vi "2_Analog_Meter_Reader(Evaluation).vi"() -> ()   [LabVIEW 2020]
uses:
  Controls/Regression_Report.ctl
  <vilib>/Ngene/DeepLTK/Toolkit/NN_Network/Controls/NN_Save_Before_Destroy_Options.ctl
  <vilib>/Ngene/DeepLTK/Toolkit/NN_Network/subVIs/NN_Predict/NN_Predict(In3D_Out1D).vi
  <vilib>/Ngene/DeepLTK/Toolkit/NN_Train/Eval_Loss/NN_Eval_Test_Error_Loss/NN_Eval(In3D_Out1D).vi
  <vilib>/Ngene/DeepLTK/Toolkit/Deep_Learning_Toolkit_by_Ngene.lvlib
panel:
  in  "Image Folder(Test)":path=path "D:/DeepLTK_Examples/Analog_Meter/Test/Images"
  in  "Labels (Test)":path=path "D:/DeepLTK_Examples/Analog_Meter/Test/Labels.csv"
  in  "NN Device":enum16{"CPU", "GPU"}(ring)=enum."GPU"
  in  "Image Folder(Train)":path=path "D:/DeepLTK_Examples/Analog_Meter/Train/Images"
  in  "Labels (Train)":path=path "D:/DeepLTK_Examples/Analog_Meter/Train/Labels.csv"
  out "Metrics (Test)":T1={"Graphs"=[{"Best Linear Fit"=[0.0, 0.7035179734230042, 1.407034993171692, 2.110553026199341, 2.814069986343384, 3.517587900161743, 4.221106052398682, 4.924623012542725, 5.628140926361084, 6.331657886505127, 7.035175800323486, 7.7386932373046875, 8.442211151123047, 9.145729064941406, 9.84924602508545, 10.552763938903809, 11.256280899047852, 11.959798812866211, 12.66331672668457, 13.366833686828613, 14.070351600646973, 14.773868560791016, 15.477387428283691, 16.180904388427734, 16.884422302246094, 17.587940216064453, 18.29145622253418, 18.99497413635254, 19.6984920501709, 20.402009963989258, 21.105527877807617, 21.809045791625977, 22.512563705444336, 23.216079711914062, 23.919597625732422, 24.62311553955078, 25.32663345336914, 26.0301513671875, 26.733667373657227, 27.437185287475586, 28.140703201293945, 28.844221115112305, 29.547739028930664, 30.251256942749023, 30.954774856567383, 31.65829086303711, 32.36180877685547, 33.06532669067383, 33.76884460449219, 34.47236251831055, 35.175880432128906, 35.879398345947266, 36.582916259765625, 37.28643035888672, 37.98994827270508, 38.69346618652344, 39.3969841003418, 40.100502014160156, 40.804019927978516, 41.507537841796875, 42.211055755615234, 42.914573669433594, 43.61809158325195, 44.32160949707031, 45.02512741088867, 45.728641510009766, 46.432159423828125, 47.135677337646484, 47.839195251464844, 48.5427131652832, 49.24623107910156, 49.94974899291992, 50.65326690673828, 51.35678482055664, 52.060302734375, 52.76382064819336, 53.46733856201172, 54.17085266113281, 54.87437057495117, 55.57788848876953, 56.28140640258789, 56.98492431640625, 57.68844223022461, 58.39196014404297, 59.09547805786133, 59.79899597167969, 60.50251388549805, 61.206031799316406, 61.909549713134766, 62.61306381225586, 63.31658172607422, 64.02010345458984, 64.72361755371094, 65.42713928222656, 66.13065338134766, 66.83416748046875, 67.53768920898438, 68.24120330810547, 68.9447250366211, 69.64823913574219, 70.35176086425781, 71.0552749633789, 71.75879669189453, 72.46231079101562, 73.16583251953125, 73.86934661865234, 74.57286071777344, 75.27638244628906, 75.97989654541016, 76.68341827392578, 77.38693237304688, 78.0904541015625, 78.7939682006836, 79.49748992919922, 80.20100402832031, 80.90452575683594, 81.60803985595703, 82.31156158447266, 83.01507568359375, 83.71858978271484, 84.42211151123047, 85.12562561035156, 85.82914733886719, 86.53266143798828, 87.2361831665039, 87.939697265625, 88.64321899414062, 89.34673309326172, 90.05024719238281, 90.75376892089844, 91.45728302001953, 92.16080474853516, 92.86431884765625, 93.56784057617188, 94.27135467529297, 94.9748764038086, 95.67839050292969, 96.38191223144531, 97.0854263305664, 97.78894805908203, 98.49246215820312, 99.19597625732422, 99.89949798583984, 100.60301208496094, 101.30653381347656, 102.01004791259766, 102.71356964111328, 103.41708374023438, 104.12060546875, 104.8241195678711, 105.52764129638672, 106.23115539550781, 106.9346694946289, 107.63819122314453, 108.34170532226562, 109.04522705078125, 109.74874114990234, 110.45226287841797, 111.15577697753906, 111.85929870605469, 112.56281280517578, 113.2663345336914, 113.9698486328125, 114.67337036132812, 115.37688446044922, 116.08039855957031, 116.78392028808594, 117.48743438720703, 118.19095611572266, 118.89447021484375, 119.59799194335938, 120.30150604248047, 121.0050277709961, 121.70854187011719, 122.41206359863281, 123.1155776977539, 123.819091796875, 124.52261352539062, 125.22612762451172, 125.92964935302734, 126.63316345214844, 127.33668518066406, 128.0402069091797, 128.74371337890625, 129.44723510742188, 130.1507568359375, 130.85427856445312, 131.5577850341797, 132.2613067626953, 132.96482849121094, 133.6683349609375, 134.37185668945312, 135.07537841796875, 135.77890014648438, 136.48240661621094, 137.18592834472656, 137.8894500732422, 138.5929718017578, 139.29647827148438, 140.0], "Array 3"=[1.1191103, 1.1208215, 2.0494566, 2.6667647, 3.113812, 4.3983607, 4.9721265, 5.639334, 6.3064847, 6.8345547, 7.8277693, 8.990467, 9.59511, 9.686706, 10.213453, 11.142547, 11.742723, 12.225249, 13.245596, 14.0788765, 14.814651, 15.36693, 15.76402, 16.432852, 17.134659, 17.87731, 18.427813, 19.16861, 20.000216, 20.941538, 21.51821, 22.116674, 22.470608, 23.3825, 24.453438, 25.066845, 25.64973, 26.13289, 26.796333, 27.819569, 28.452826, 29.007662, 29.715298, 30.633392, 31.342394, 32.035053, 32.61452, 33.464294, 34.276417, 34.943382, 35.97995, 36.556244, 37.02365, 37.705124, 38.3015, 39.360004, 39.889103, 40.30833, 40.943993, 41.4772, 42.169846, 42.81026, 43.799282, 44.6952, 45.416332, 46.042446, 46.79732, 47.508343, 48.09876, 48.742836, 49.218735, 49.851227, 50.669456, 51.317608, 51.95643, 52.556763, 53.286587, 53.868534, 54.71111, 55.695065, 56.496944, 57.143272, 57.87432, 58.363266, 59.263767, 59.95194, 60.54199, 61.248116, 62.144474, 62.750816, 63.315197, 63.991894, 64.673294, 65.21437, 65.78511, 66.731705, 67.40204, 68.17529, 68.910904, 69.6694, 70.56884, 71.38461, 72.153244, 72.770386, 73.40299, 73.98696, 74.56206, 75.30551, 76.02788, 76.8059, 77.393326, 78.05725, 78.863556, 79.64017, 80.19238, 80.80632, 81.75397, 82.49788, 83.45299, 83.8592, 84.582375, 85.37528, 86.09314, 86.848175, 87.40028, 88.08168, 88.83669, 89.5325, 90.27479, 90.954704, 91.40349, 91.8369, 92.65036, 93.7729, 94.60417, 95.43445, 96.11843, 96.73094, 97.527145, 98.015366, 98.69766, 99.33419, 99.997765, 100.65184, 101.144066, 102.21565, 102.77403, 103.49586, 103.97933, 104.69403, 105.7315, 106.22682, 106.847534, 107.528824, 108.24076, 108.93027, 109.59428, 110.28842, 110.89985, 111.587975, 112.43388, 113.592705, 114.30132, 114.76443, 115.22754, 115.85933, 117.078224, 118.21052, 118.373405, 118.85284, 119.099075, 120.0473, 120.72142, 121.46607, 122.0247, 122.7984, 123.476135, 124.20413, 124.859024, 125.31311, 125.978096, 126.854614, 127.88554, 128.6452, 129.04144, 129.79903, 130.51143, 130.49928, 131.18375, 132.28572, 133.07285, 133.94731, 134.7844, 135.33304, 136.06282, 136.96729, 137.98709, 138.17464, 138.51686, 138.61647]}, {"Best Linear Fit"=[0.5510894536551477, 0.5528118856345293, 1.4875805447104122, 2.1089659407688175, 2.558965874975776, 3.851998945803168, 4.4295543638213815, 5.101168919513712, 5.77272587681186, 6.304283697222128, 7.304058383959592, 8.47443567437423, 9.083072145866842, 9.17527277535532, 9.705499592873341, 10.640729519089307, 11.244870435915933, 11.73058329446284, 12.757669219775421, 13.59645351485162, 14.337087266320234, 14.893014487322722, 15.292727183514954, 15.965976573628847, 16.67241895833718, 17.419975076813355, 17.97411386767646, 18.719803798181108, 19.556902380254215, 20.50444204328033, 21.084922499749805, 21.687340264617124, 22.043611291943282, 22.96152618089459, 24.039537726424093, 24.656996351959073, 25.243731994036825, 25.730083234785926, 26.397907816141014, 27.427901500386604, 28.065341008863673, 28.623841918112905, 29.336151659242017, 30.260310214122768, 30.973994636926378, 31.671228958351318, 32.254524056349865, 33.10991012857609, 33.92739645742988, 34.598767179920166, 35.6421812900104, 36.222281597078265, 36.69277599990878, 37.37874983527094, 37.9790633388041, 39.044560673224105, 39.577153824769816, 39.99915037969822, 40.63901094067745, 41.1757396569255, 41.87296053872513, 42.5176056063145, 43.51315929073158, 44.41499654791994, 45.14088991034388, 45.771139219280435, 46.53100027470058, 47.24671792081885, 47.84103351157109, 48.48936487638817, 48.968406880915445, 49.60507649085694, 50.428710488316526, 51.08114285879944, 51.72418285113757, 52.328482163548195, 53.06312664199501, 53.64891767040816, 54.49705786464616, 55.48751217123157, 56.2946883875266, 56.94528528918154, 57.681162373263874, 58.17333681166488, 59.07978578028082, 59.77250246765534, 60.36644942868481, 61.07724049215396, 61.97951933703106, 62.5898664808309, 63.15797480222986, 63.839141091624214, 64.5250419690204, 65.06969238441509, 65.64420180735426, 66.59704820243111, 67.2718095503923, 68.05017121002403, 68.79064080606922, 69.55414975978763, 70.45952739827176, 71.28068850467443, 72.05439621405617, 72.67561409478483, 73.31239890151468, 73.90022507318898, 74.47911965387195, 75.22748406981316, 75.95462155755145, 76.7377830833651, 77.32908819804804, 77.99739852586073, 78.80902901797258, 79.59076978339638, 80.14663268619204, 80.76462505684644, 81.71853126237625, 82.46735646547093, 83.42877350160221, 83.83766834180045, 84.5656198868432, 85.36376467493032, 86.086363409207, 86.84638574013086, 87.40214112592403, 88.08803816342727, 88.84803745499346, 89.54844160804494, 90.29563101674482, 90.9800381757852, 91.4317862212556, 91.86805949815552, 92.68689362943319, 93.8168512467299, 94.65360999827732, 95.48937037765891, 96.17787086257923, 96.79442711327201, 97.59588956886408, 98.08733442760543, 98.77413767984383, 99.4148698965217, 100.0828269541834, 100.74122267841074, 101.2366994247449, 102.31536375207514, 102.87743192187078, 103.60402414481081, 104.09069217672791, 104.81011147964568, 105.85443180447106, 106.35302654387701, 106.97783856440267, 107.66362808490345, 108.38026730532866, 109.07432795523411, 109.7427227606916, 110.44145272041884, 111.05691844151508, 111.74958905017425, 112.60108531084664, 113.76756031005539, 114.48085882361796, 114.94702182720592, 115.41319251057976, 116.04915558021928, 117.2761012135343, 118.41587359719979, 118.57983702597413, 119.06243477136897, 119.31029986100326, 120.26478973026079, 120.94336025202396, 121.69293039435007, 122.25524431729423, 123.03405908429353, 123.71626982456907, 124.44907499429496, 125.10829245561264, 125.56537795227734, 126.2347557703289, 127.11706333199626, 128.1547944005271, 128.91947836148685, 129.31833572152544, 130.08092310093693, 130.79803078830147, 130.7858045691629, 131.47478888059436, 132.58404179512874, 133.37636530551043, 134.25660700477312, 135.0992177531695, 135.65148651616815, 136.38608875579257, 137.29652737317892, 138.32306899366648, 138.51185349044076, 138.8563379663706, 138.9566052509644], "Array 3"=[1.1191103, 1.1208215, 2.0494566, 2.6667647, 3.113812, 4.3983607, 4.9721265, 5.639334, 6.3064847, 6.8345547, 7.8277693, 8.990467, 9.59511, 9.686706, 10.213453, 11.142547, 11.742723, 12.225249, 13.245596, 14.0788765, 14.814651, 15.36693, 15.76402, 16.432852, 17.134659, 17.87731, 18.427813, 19.16861, 20.000216, 20.941538, 21.51821, 22.116674, 22.470608, 23.3825, 24.453438, 25.066845, 25.64973, 26.13289, 26.796333, 27.819569, 28.452826, 29.007662, 29.715298, 30.633392, 31.342394, 32.035053, 32.61452, 33.464294, 34.276417, 34.943382, 35.97995, 36.556244, 37.02365, 37.705124, 38.3015, 39.360004, 39.889103, 40.30833, 40.943993, 41.4772, 42.169846, 42.81026, 43.799282, 44.6952, 45.416332, 46.042446, 46.79732, 47.508343, 48.09876, 48.742836, 49.218735, 49.851227, 50.669456, 51.317608, 51.95643, 52.556763, 53.286587, 53.868534, 54.71111, 55.695065, 56.496944, 57.143272, 57.87432, 58.363266, 59.263767, 59.95194, 60.54199, 61.248116, 62.144474, 62.750816, 63.315197, 63.991894, 64.673294, 65.21437, 65.78511, 66.731705, 67.40204, 68.17529, 68.910904, 69.6694, 70.56884, 71.38461, 72.153244, 72.770386, 73.40299, 73.98696, 74.56206, 75.30551, 76.02788, 76.8059, 77.393326, 78.05725, 78.863556, 79.64017, 80.19238, 80.80632, 81.75397, 82.49788, 83.45299, 83.8592, 84.582375, 85.37528, 86.09314, 86.848175, 87.40028, 88.08168, 88.83669, 89.5325, 90.27479, 90.954704, 91.40349, 91.8369, 92.65036, 93.7729, 94.60417, 95.43445, 96.11843, 96.73094, 97.527145, 98.015366, 98.69766, 99.33419, 99.997765, 100.65184, 101.144066, 102.21565, 102.77403, 103.49586, 103.97933, 104.69403, 105.7315, 106.22682, 106.847534, 107.528824, 108.24076, 108.93027, 109.59428, 110.28842, 110.89985, 111.587975, 112.43388, 113.592705, 114.30132, 114.76443, 115.22754, 115.85933, 117.078224, 118.21052, 118.373405, 118.85284, 119.099075, 120.0473, 120.72142, 121.46607, 122.0247, 122.7984, 123.476135, 124.20413, 124.859024, 125.31311, 125.978096, 126.854614, 127.88554, 128.6452, 129.04144, 129.79903, 130.51143, 130.49928, 131.18375, 132.28572, 133.07285, 133.94731, 134.7844, 135.33304, 136.06282, 136.96729, 137.98709, 138.17464, 138.51686, 138.61647]}, {"Best Linear Fit"=[0.0, 140.0], "Array 3"=[0.0, 140.0]}], "y=k*x+b"="y = 0.993*x + 0.572", "R"=0.99997884, "R^2"=0.9999577, "MAE"=0.30468705, "MSE"=0.1540845} {"R" format="%#_7g"}
  out "Metrics (Train)":T1={"Graphs"=[{"Best Linear Fit"=array[1000 elements], "Array 3"=array[1000 elements]}, {"Best Linear Fit"=array[1000 elements], "Array 3"=array[1000 elements]}, {"Best Linear Fit"=[0.0, 140.0], "Array 3"=[0.0, 140.0]}], "y=k*x+b"="y = 0.994*x + 0.559", "R"=0.9999774, "R^2"=0.9999548, "MAE"=0.3035189, "MSE"=0.1533813} {"R" format="%#_7g"}
  in  "Network Configuration File Path":path=path "D:/Ngene/GitHub/deepltk_examples/3_Image_Processing/31_Image_Regression/working/Analog_Meter/Analog_Meter_net_cfg_23_11_30__17_47_53.cfg"
  in  "Weight File Path":path=path "D:/Ngene/GitHub/deepltk_examples/3_Image_Processing/31_Image_Regression/working/Analog_Meter/Analog_Meter_weights_23_11_30__17_47_53.bin"
  # "Overview: Performs evaluation of a trained model over Training and Tests Datasets\nInstructions:\n1. Provide paths to Train and Test datasets \n2. Provide model files (.cfg and .bin).\n2. Run the VI\n3. Drag and drop image on \"Input Image\"\n4. Observe calculated metrics on both train and test datasets."
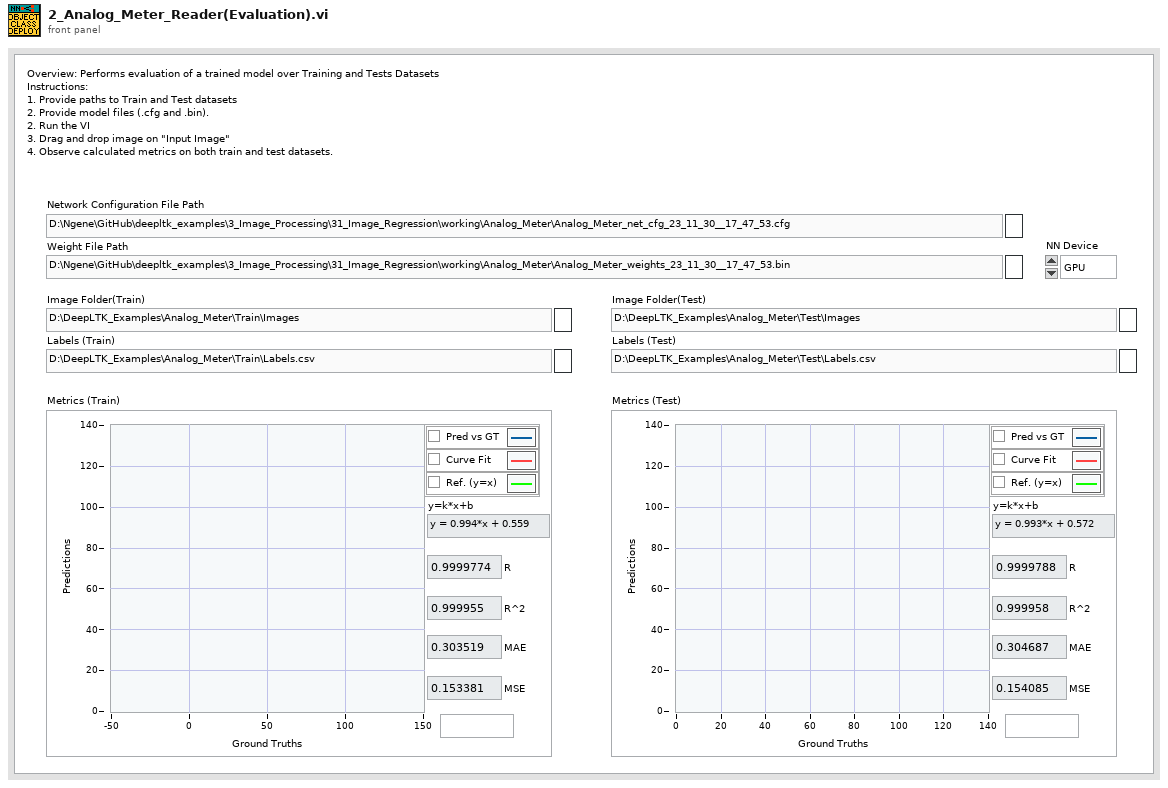
[diagram p1: front panel]
types:
  T1 = typedef "Regression_Report.ctl" = cluster{"Graphs":cluster{"Best Linear Fit":dbl[], "Array 3":sgl[]}[], "y=k*x+b":string, "R":sgl, "R^2":sgl, "MAE":sgl, "MSE":sgl}
  T2 = typedef "Deep_Learning_Toolkit_by_Ngene.lvlib/NN_Save_Before_Destroy_Options.ctl" = cluster{"CFG?":bool, "Weights?":bool, "Render?":bool}
  T3 = typedef "Deep_Learning_Toolkit_by_Ngene.lvlib/NN_Config_Params.ctl" = cluster{"Name":string, "mBatch":i32, "NN_Train_Params":T4, "LR_Decay_Policy":T7, "Labels":string[], "Loss":T9}
  T4 = typedef "Deep_Learning_Toolkit_by_Ngene.lvlib/NN_Train_Params.ctl" = cluster{"Optimizer":T5, "Beta_1":sgl, "Beta_2":sgl, "Weight Decay(L1)":sgl, "Weight Decay(L2)":sgl, "Data_Sampling":T6}
  T5 = typedef "Deep_Learning_Toolkit_by_Ngene.lvlib/NN_Train_Optimizer.ctl" = enum16{"SGD", "Adam", "Adagrad", "Adadelta", "RMSProp", "Nesterov"}
  T6 = typedef "Deep_Learning_Toolkit_by_Ngene.lvlib/NN_Train_Data_Sampling.ctl" = enum16{"Random", "Sequential"}
  T7 = typedef "Deep_Learning_Toolkit_by_Ngene.lvlib/NN_LR_Policy_Cfg.ctl" = cluster{"Policy_Type":T8, "LR0":dbl, "k":sgl, "WarmUp_Policy":enum16{"Step", "Ramp"}, "WarmUp_Iter":i32, "WarmUp_Ratio":sgl}
  T8 = typedef "Deep_Learning_Toolkit_by_Ngene.lvlib/NN_LR_Policy_Type.ctl" = enum16{"Manual", "Step", "Exp", "1/t"}
  T9 = typedef "Deep_Learning_Toolkit_by_Ngene.lvlib/NN_Loss_Config_Params.ctl" = cluster{"Loss_Type":T10, "Loss_Conf_Params":variant}
  T10 = typedef "Deep_Learning_Toolkit_by_Ngene.lvlib/NN_Loss_Type.ctl" = enum16{"None", "MSE", "CrossEntropy", "YOLO_v2"}
  T11 = typedef "Deep_Learning_Toolkit_by_Ngene.lvlib/NN_Layer_Config_Params.ctl" = cluster{"Layer_Type":T12, "Layer_Conf_Params":variant}
  T12 = typedef "Deep_Learning_Toolkit_by_Ngene.lvlib/NN_Layer_Type.ctl" = enum16{"Input1D", "Input3D", "Conv2D", "Conv2D_Adv", "MaxPool", "AvgPool", "UpSample", "DropOut3D", "ShortCut", "Concat", "SoftMax3D", "FC", "DropOut", "Softmax", "Flatten", "YOLO_v2", "Unsupported"}
  T13 = typedef "Deep_Learning_Toolkit_by_Ngene.lvlib/NN.ctl" = cluster{"Name":string, "No of Layers":i32, "mBatch":i32, "Layers":T14[], "Dimty":T15, "Dims_In":T16, "Dims_Out":T16, "Working_Dir":path, "Train?":bool, "Train_Params":T4, "LR_Update_Policy":T7, "Session Data":T17, "Ground_truth":T18, "NNg_hdls":T20, "NN_Device":T21, "GPU Id":i32, "Labels":string[], "Receptive Field":T22[], "Loss_Type":T10, "Loss_Cfg_Prms":variant}
  T14 = typedef "Deep_Learning_Toolkit_by_Ngene.lvlib/NN_Layer_ref.ctl" = refnum<data-value>
  T15 = typedef "Deep_Learning_Toolkit_by_Ngene.lvlib/NN_In_Out_Dim-ty.ctl" = enum8{"In1D_Out1D", "In3D_Out1D", "In3D_Out3D", "In3D_OutBBox"}
  T16 = typedef "Deep_Learning_Toolkit_by_Ngene.lvlib/NN_Dims(C,H,W).ctl" = cluster{"C":i32, "H":i32, "W":i32}
  T17 = typedef "Deep_Learning_Toolkit_by_Ngene.lvlib/NN_Train_Session_Data.ctl" = cluster{"Epochs":sgl, "Tot_Iter":i32, "LR":sgl, "LR_iter":i32}
  T18 = typedef "Deep_Learning_Toolkit_by_Ngene.lvlib/NN_Ground_truth.ctl" = cluster{"Y":variant, "Y_idx":T19}
  T19 = typedef "Deep_Learning_Toolkit_by_Ngene.lvlib/NN_Data_ref(1D_I32).ctl" = refnum<data-value>
  T20 = typedef "Deep_Learning_Toolkit_by_Ngene.lvlib/nng_cuda_handles.ctl" = cluster{"cudnn":u64, "cublas":u64, "stream":u64, "curand":u64}
  T21 = typedef "Deep_Learning_Toolkit_by_Ngene.lvlib/NN_Device.ctl" = enum16{"CPU", "GPU"}
  T22 = typedef "Deep_Learning_Toolkit_by_Ngene.lvlib/NN_Dims(V,H).ctl" = cluster{"V":i32, "H":i32}
  T23 = typedef "Deep_Learning_Toolkit_by_Ngene.lvlib/NN_DataSets_All(In3D_Out1D).ctl" = cluster{"Train":T24, "Validation":T24, "Test":T24}
  T24 = typedef "Deep_Learning_Toolkit_by_Ngene.lvlib/NN_DataSet(In3D_Out1D).ctl" = cluster{"Inputs Ref.":T25, "Outputs Ref.":T26, "Dataset_Size":i32, "Outputs_idx Ref.":T19, "Dims_In":T16, "Dims_Out":i32, "Labels":string[], "File Paths":path[]}
  T25 = typedef "Deep_Learning_Toolkit_by_Ngene.lvlib/NN_Data_ref(4D_SGL).ctl" = refnum<data-value>
  T26 = typedef "Deep_Learning_Toolkit_by_Ngene.lvlib/NN_Data_ref(2D_SGL).ctl" = refnum<data-value>
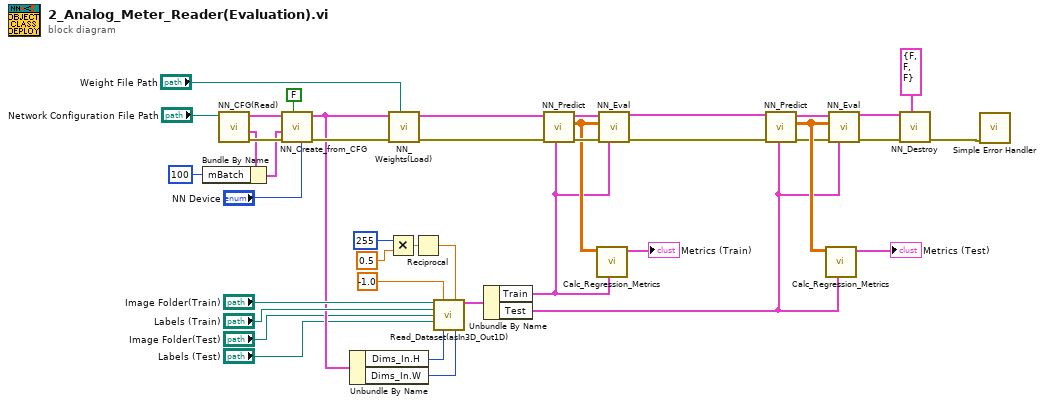
[diagram p0: block diagram]
diagram:
  n1 = call <vilib>:"NN_CFG(Read).vi"("CFG file path"="Network Configuration File Path") -> ("error out"=w41:errorcluster, "Net_Cfg"=w35:T3, "Layer_Cfg"=w34:T11[])  [unwired: 8 in]
  n2 = Bundle By Name(cluster=w35, "mBatch"=100) -> (w32:T3)
  n3 = call <vilib>:"NN_Create_from_CFG.vi"("NN_Device"="NN Device", "Train? (false)"=FALSE, "error in (no error)"=w41, "Net_Cfg"=w32, "Layer_Cfg"=w34) -> ("error out"=w37:errorcluster, "NN out"=w9:T13)  [unwired: 5 in]
  n4 = Unbundle By Name(w9) -> ("Dims_In.H"=w8:i32, "Dims_In.W"=w7:i32)
  n5 = Multiply(x=u16 255 ("Shift"), y=sgl 0.5 ("Scale")) -> (x*y=w27:sgl)
  n6 = call <vilib>:"NN_Weights(Load).vi"("Weight File Path"="Weight File Path", "error in (no error)"=w37, "NN in"=w9) -> ("error out"=w21:errorcluster, "NN out"=w33:T13)  [unwired: 7 in]
  n7 = Reciprocal(x=w27) -> (1/x=w26:sgl)
  n8 = call "Read_Dataset(asIn3D_Out1D).vi"("Image Folder Path(Train)"="Image Folder(Train)", "Norm. Shift"=sgl -1.0 ("Scale"), "Norm. Scale"=w26, "Label File Path(Train)"="Labels (Train)", "Image Folder Path(Test)"="Image Folder(Test)", "Label File Path(Test)"="Labels (Test)", "Img Heigth"=w8, "Img Width"=w7) -> ("Datasets"=w22:T23)  [unwired: 6 in, 1 out]
  n9 = Unbundle By Name(w22) -> ("Train"=w6:T24, "Test"=w5:T24)
  n10 = call-poly <vilib>:"NN_Predict.vi"("Dataset"=w6, "error in (no error)"=w21, "NN in"=w33) -> ("error out"=w24:errorcluster, "Predictions"=w23:sgl[][], "NN out"=w25:T13)  [unwired: 6 in]
  n11 = call "Calc_Regression_Metrics.vi"("Dataset"=w6, "Predictions"=w23) -> ("Metrics"=→"Metrics (Train)":T1)  [unwired: 9 in]
  n12 = call-poly <vilib>:"NN_Eval.vi"("NN in"=w25, "Predictions"=w23, "error in (no error)"=w24, "Dataset"=w6) -> ("NN out"=w17:T13, "error out"=w16:errorcluster)  [unwired: 7 in, 3 out]
  n13 = call-poly <vilib>:"NN_Predict.vi"("Dataset"=w5, "error in (no error)"=w16, "NN in"=w17) -> ("error out"=w19:errorcluster, "Predictions"=w20:sgl[][], "NN out"=w18:T13)  [unwired: 6 in]
  n14 = call "Calc_Regression_Metrics.vi"("Dataset"=w5, "Predictions"=w20) -> ("Metrics"=→"Metrics (Test)":T1)  [unwired: 9 in]
  n15 = call-poly <vilib>:"NN_Eval.vi"("NN in"=w18, "Predictions"=w20, "error in (no error)"=w19, "Dataset"=w5) -> ("NN out"=w15:T13, "error out"=w14:errorcluster)  [unwired: 7 in, 3 out]
  n16 = call <vilib>:"NN_Destroy.vi"("Save (T, T, T)"=T2 {"CFG?"=FALSE, "Weights?"=FALSE, "Render?"=FALSE} ("Save_Config"), "error in (no error)"=w14, "NN in"=w15) -> ("error out"=w39:errorcluster)  [unwired: 8 in]
  n17 = call <vilib>:"Simple Error Handler.vi"("error in (no error)"=w39) -> ()  [unwired: 4 in, 5 out]
